vi "WordE.vi"() -> ()   [LabVIEW 2018]
uses:
  <vilib>/Utility/file.llb/Read Delimited Spreadsheet (DBL).vi
panel:
  out "all rows":dbl[][](array[numeric])=[[-3.0, 2.5, -0.75], [-2.99816, 2.502, -0.75116], [-2.99244, 2.50791, -0.75467], [-2.98223, 2.51745, -0.76053], [-2.96644, 2.53014, -0.76879], [-2.94347, 2.54525, -0.77951], [-2.91108, 2.56174, -0.79277], [-2.86629, 2.57821, -0.80868], [-2.80538, 2.59277, -0.82736], [-2.72404, 2.60308, -0.84901], [-2.61849, 2.60628, -0.87371], [-2.49528, 2.60021, -0.89977], [-2.35932, 2.58465, -0.92672], [-2.21416, 2.55992, -0.95466], [-2.06363, 2.52652, -0.98376], [-1.9113, 2.48507, -1.01419], [-1.75999, 2.43616, -1.04619], [-1.61162, 2.38022, -1.08006], [-1.4672, 2.31748, -1.11624], [-1.32687, 2.24788, -1.15531], [-1.19319, 2.1728, -1.19717], [-1.07471, 2.09843, -1.23909], [-0.97029, 2.02629, -1.28087], [-0.87834, 1.95735, -1.32252], [-0.7976, 1.89248, -1.36406], [-0.72714, 1.83257, -1.40552], [-0.66633, 1.77846, -1.4469], [-0.61473, 1.73105, -1.48823], [-0.57209, 1.69124, -1.52952], [-0.53828, 1.65992, -1.57079], [-0.53828, 1.65992, -1.57079], [-0.54414, 1.67596, -1.5708], [-0.56114, 1.72333, -1.5708], [-0.58748, 1.79988, -1.5708], [-0.61585, 1.88822, -1.5708], [-0.64068, 1.97318, -1.5708], [-0.6618, 2.05515, -1.5708], [-0.67639, 2.12137, -1.5708], [-0.68373, 2.16024, -1.5708], [-0.68592, 2.17306, -1.5708], [-0.68592, 2.17306, -1.5708], [-0.70868, 2.18105, -1.5708], [-0.7772, 2.20247, -1.5708], [-0.89141, 2.22935, -1.5708], [-1.02597, 2.24643, -1.5708], [-1.154, 2.24643, -1.5708], [-1.27138, 2.22935, -1.5708], [-1.35855, 2.20247, -1.5708], [-1.40554, 2.18105, -1.5708], [-1.42027, 2.17306, -1.5708], [-1.42027, 2.17306, -1.5708], [-1.40959, 2.16025, -1.57079], [-1.37786, 2.12137, -1.57079], [-1.32593, 2.05515, -1.57079], [-1.26477, 1.97319, -1.57079], [-1.20433, 1.88822, -1.57079], [-1.14408, 1.79989, -1.57079], [-1.09365, 1.72334, -1.57079], [-1.06315, 1.67597, -1.57079], [-1.05293, 1.65992, -1.57079], [-1.05293, 1.65992, -1.57079], [-1.05293, 1.65992, -1.56133], [-1.05293, 1.65992, -1.50808], [-1.05293, 1.65992, -1.39853], [-1.05293, 1.65992, -1.24519], [-1.05293, 1.65992, -1.0756], [-1.05293, 1.65992, -0.92227], [-1.05293, 1.65992, -0.81272], [-1.05293, 1.65992, -0.75947], [-1.05293, 1.65992, -0.75], [-1.05293, 1.65992, -0.75], [-1.05799, 1.67945, -0.75], [-1.07195, 1.73674, -0.75], [-1.09104, 1.82813, -0.75], [-1.10688, 1.93174, -0.75], [-1.11452, 2.02934, -0.75], [-1.11307, 2.12127, -0.75], [-1.10404, 2.19359, -0.75], [-1.09482, 2.23508, -0.75], [-1.09106, 2.24858, -0.75], [-1.09106, 2.24858, -0.75], [-1.09106, 2.24858, -0.75947], [-1.09106, 2.24858, -0.81272], [-1.09106, 2.24858, -0.92227], [-1.09106, 2.24858, -1.0756], [-1.09106, 2.24858, -1.24519], [-1.09106, 2.24858, -1.39853], [-1.09106, 2.24858, -1.50808], [-1.09106, 2.24858, -1.56133], [-1.09106, 2.24858, -1.57079], [-1.09107, 2.24858, -1.5708], [-1.08431, 2.23514, -1.57079], [-1.06389, 2.19452, -1.57079], [-1.02933, 2.12576, -1.57079], [-0.98692, 2.0413, -1.57079], [-0.9433, 1.95441, -1.57079], [-0.89828, 1.86468, -1.57079], [-0.85951, 1.78737, -1.57079], [-0.83562, 1.73973, -1.57079], [-0.82754, 1.72362, -1.57079], [-0.82754, 1.72362, -1.57079], [-0.82754, 1.72362, -1.56133], [-0.82754, 1.72362, -1.50807], [-0.82754, 1.72362, -1.39853], [-0.82754, 1.72362, -1.24519], [-0.82754, 1.72362, -1.0756], [-0.82754, 1.72362, -0.92226], [-0.82754, 1.72362, -0.81272], [-0.82754, 1.72362, -0.75947], [-0.82754, 1.72362, -0.75], [-0.82754, 1.72362, -0.75], [-0.82838, 1.72392, -0.75], [-0.83395, 1.72591, -0.75], [-0.84801, 1.73094, -0.75], [-0.8734, 1.74001, -0.75], [-0.91207, 1.75383, -0.75], [-0.96517, 1.77281, -0.75], [-1.03313, 1.79709, -0.75], [-1.11571, 1.82661, -0.75], [-1.21214, 1.86107, -0.75], [-1.32111, 1.90001, -0.75], [-1.44092, 1.94283, -0.75], [-1.56951, 1.98878, -0.75], [-1.70458, 2.03705, -0.75], [-1.8436, 2.08673, -0.75], [-1.98394, 2.13689, -0.75], [-2.12296, 2.18657, -0.75], [-2.25802, 2.23484, -0.75], [-2.38662, 2.2808, -0.75], [-2.50643, 2.32361, -0.75], [-2.6154, 2.36256, -0.75], [-2.71183, 2.39701, -0.75], [-2.79441, 2.42653, -0.75], [-2.86237, 2.45081, -0.75], [-2.91547, 2.46979, -0.75], [-2.95414, 2.48361, -0.75], [-2.97953, 2.49268, -0.75], [-2.99359, 2.49771, -0.75], [-2.99915, 2.4997, -0.75], [-3.0, 2.5, -0.75]]
  in  "file path (dialog if empty)":path=path "/Users/JoshEtkind/Documents/Tufts/Senior Fall/Advanced Robotics/Initials/Physical Robot/wordE.csv"
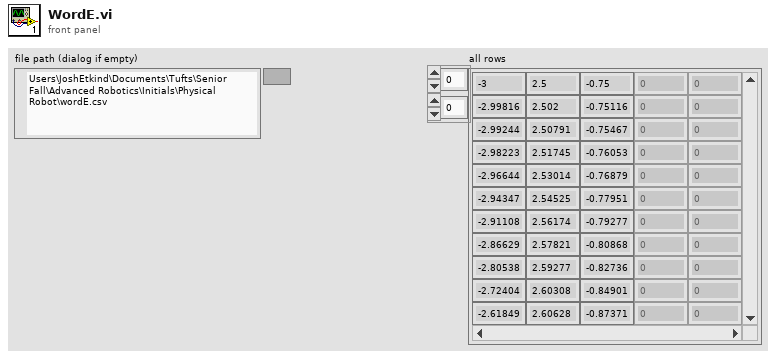
[diagram p1: front panel]
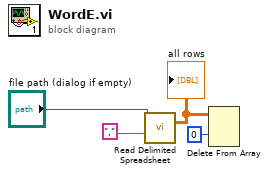
[diagram p0: block diagram]
diagram:
  n1 = call-poly <vilib>:"Read Delimited Spreadsheet.vi"("file path (dialog if empty)"="file path (dialog if empty)", "delimiter (\\t)"="," ("delimiter (\\t)")) -> ("all rows"=w2:dbl[][])  [unwired: 8 in, 5 out]
  "all rows" <- w2
  n2 = Delete From Array(array=w2, index (row)=0) -> ()  [unwired: 2 in, 2 out]
